vi "ROI Entry Screen_v3.vi"() -> ()   [LabVIEW 2020]
uses:
  Typedefs/Top level VI states.ctl
  ROI Entry screen/Typedefs/ROI move buttons.ctl
  ROI Entry screen/Typedefs/ROI move mode.ctl
  Typedefs/Offsets cluster.ctl
  ROI Entry screen/Typedefs/FGV ROI Time Ops.ctl
  Typedefs/ROI management FG states.ctl
  ROI Entry screen/Typedefs/Redraw ROI.ctl
  ROI Entry screen/Typedefs/ROI Lbox actions.ctl
  ROI Entry screen/SubVIs/Automatic POI detection/Typedefs/Duplicate POI function enum.ctl
  Typedefs/Read Write Enum.ctl
  ROI Entry screen/Typedefs/ROI entry screen ctrl refs cluster.ctl
  Global Variables/General Globals.vi
  User profiles code/Globals/gl_UsrProfiles globals.vi
  ROI Entry screen/Globals/gl_ROI Entry UI globals.vi
  ROI Entry screen/Typedefs/ROI input mode.ctl
panel:
  out "ROI Type":string
  out "Array":bool[](array[boolean])
  in  "Offset ROI":bool
  in  "Arbitrary Plane":bool
  in  "Whole Plane":bool
  in  "Equal Size":bool
  in  "Line Mode":bool
  out "Current ROI Type":string
  out "AOL Z ind. (um)":dbl caption="Motor Z" format="AOL Z   =  %#_g µm"
  in  "Load Reference Image":bool
  out "# POI":i32 format="%.0f ROI"
  in  "Max Z Proj":bool
  out "ROI":T1
  out "Number of lines left":i32 format="%.0f number of lines left"
  in  "Palette Type":T2(ring)
  out "Zplane ind":i32 caption="Z-Plane" format="Z-Plane %.0f"
  in  "Z-Plane Selector":i32(c297)=7
  out "Image Display":T3(plugin-control)
  out "Motor Z ind. (um)":dbl caption="Motor Z" format="Motor Z = %#_g µm"
  out "# of planes":i32 format="# of Planes = %.0f"
  in  "Intensity slider":cluster{i16, i16}(slide)={0, 4095} caption="Intensity" scale=0.0..4095.0
  in  "Channel":enum16{"Green", "Red"}(ring)
  in  "Step size (µm)":u8(slide)=1 min=1 max=100 step=1 scale=1.0..30.0
  in  "ROI offset arrows":T4
  in  "ROI move mode":T5
  in  "Auto Generate":bool
  in  "POI Density":dbl(slide) scale=0.01..1.0
  in  "Tab Control":enum32{"ROI Details", "Folder", "Vaa3D"}(tab)
  in  "Adj. \nMC":bool
  out "Dwell Time (Ind.)":dbl caption="Dwell Time" format="%.2f us"
  out "Laser Power (Ind.)":dbl caption="Laser Power" format="%u %"
  out "Pixel Density (Ind.)":dbl caption="Pixel Density" format="%.2f px/um"
  out "Cycle rate":dbl format="%.2f Hz"
  out "Resolution (Ind.)":dbl caption="Resolution" format="%.2f um/px"
  in  "Laser Power(%)":dbl min=0.0 max=100.0 step=1.0
  in  "Show All":bool
  in  "Delete Lines":bool
  in  "Save ROI File":bool
  in  "ROI LIST":i32[](listbox)
  in  "Rel.  Res.":dbl=1.0 format="%.2g"
  in  "Funct stim.trig.delay (sec)":dbl=0.5 caption="Stimulus trigger delay" min=0.0 max=60.0 step=0.001 format="%#.3fs"
  in  "Enable funct. stimulus":bool caption="Enable stimulus"
  in  "Wavelength (nm)":dbl=920.0 caption="l" min=800.0 max=1080.0 step=1.0 format="%#_g nm"
  in  "Number of Trials":u16=1 caption="Trials" min=1 max=1000 format="%.0f trials"
  in  "Dwell time [us]":dbl=0.1 caption="Scan dwell time\nper pixel (us)" min=0.05 max=20.0 step=0.01 format="%.2f"
  in  "POI dwell time (us)":dbl=4.0 caption="POI dwell time" min=0.05 max=20.0 format="%_3g µs"
  in  "Zoom":dbl=1.0 min=0.001 max=10.0 step=0.1 format="%#.2f x"
  in  "Trial Length (sec)":dbl=1.0 caption="Trial Length" min=0.05 max=60.0 step=1.0 format="%#.3f s"
  in  "Cool-down time (s)":dbl caption="Cool-down time" min=0.0 max=60.0 step=0.05 format="%#.2f s"
  in  "Enable cool-down time":bool caption="Enable stimulus"
  in  "Load ROI File":bool caption="Load\nolder\nPOI"
  in  "Start Plane":i32 caption="From Plane"
  in  "Stop Plane":i32 caption="To Plane"
  in  "Clear All":bool
  in  "Clear Last":bool
  out "Frame Size (Ind.)":dbl caption="Frame Size"
  out "FOV (Ind.)":dbl caption="FOV" format="%d um"
  out "ZPlanes":dbl[][](array[numeric])
  in  "Z-stack folder path":path caption="Experiment folder path"
  in  "spacing_between_points":dbl=10.0 min=0.05 max=100.0 step=1.0 format="%#.3f"
  in  "Call_Vaa3D":bool caption="Load\nolder\nPOI"
  out "Next State":T6=enum."Live Imaging-START"
  in  "Live Imaging":bool
  in  "Acquisition":bool
  in  "Done/Close":bool
  # "ROI Offset"
  # "ROI Removal"
  # "ROI Input"
  # "ROI AutoGen"
  # "Min"
  # "Max"
  # "Plane Filter :"
  # "Original Z Stack Settings"
  # "ROI Input Settings"
  # "Stimulus trigger delay"
  # "Experiment Settings"
  # "Cool-down time"
  # "AOLZ"
  # "Motor Z"
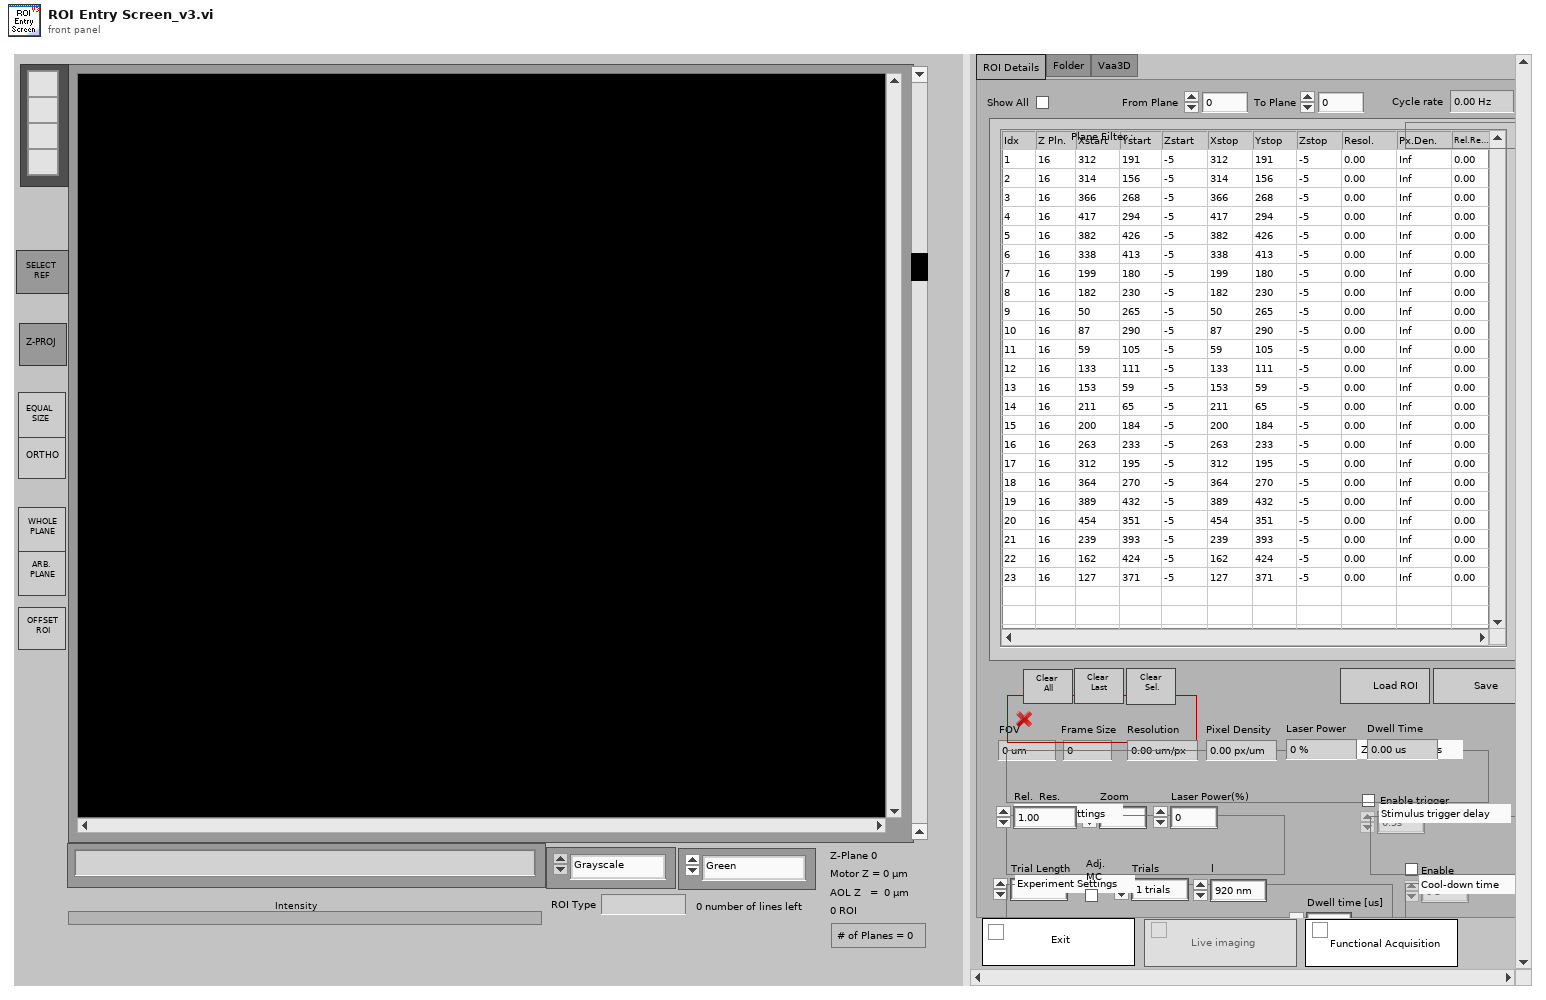
[diagram p1: front panel]
types:
  T1 = cluster{"Global Rectangle":i32[], "Contours":cluster{"Contour Type":u32, "ROI Type":u32, "Points":i32[]}[]}
  T2 = enum16{"Grayscale", "Binary", "Gradient", "Rainbow", "Temperature", "User Defined"}
  T3 = typedef "IMAQ Image.ctl" = refnum<image>
  T4 = typedef "ROI move buttons.ctl" = cluster{"Right":bool, "Left":bool, "Up":bool, "Down":bool, "Up-left":bool, "Up-right":bool, "Down-left":bool, "Down-right":bool}
  T5 = typedef "ROI move mode.ctl" = enum16{"ROI on ALL planes", "ROI on current plane"}
  T6 = typedef "Top level VI states.ctl" = enum16{"None", "Initialise UI", "<STACK PROTOCOL STATES>", "AOL Zstack-START", "AOL Zstack-STOP", "Motor Zstack-START", "Motor Zstack-STOP", "Parameter Sweep-START", "Parameter Sweep-STOP", "<ACQUISITION PROTOCOL STATES> ", "Functional Acquisition-START", "Functional Acquisition-STOP", "Single Plane Acquisition-START", "Single Plane Acquisition-STOP", "Volume Acquisition-START", "Volume Acquisition-STOP", "<LIVE IMAGING PROTOCOL STATES>", "Live Imaging-START", "Live Imaging-STOP", "Live Plane Imaging-START", "Live Plane Imaging-STOP", "Live Volume Imaging-START", "Live Volume Imaging-STOP", "<MOVEMENT CORRECTION PROTOCOL STATES>", "EXIT"}
  T7 = typedef "Offsets cluster.ctl" = cluster{"X offset":i8, "Y offset":i8}
  T8 = cluster{"Load experiment data":refnum<user-event>, "Finish rectangle editing":refnum<user-event>, "Offset all ROI":refnum<user-event>}
  T9 = typedef "ROI info cluster.ctl" = cluster{"Global Rectangle":i32[], "Contours":cluster{"Contour Type":u32, "ROI Type":u32, "Points":i32[]}[]}
  T10 = typedef "FGV ROI Time Ops.ctl" = enum16{"Read", "Write Cycle Time", "Write Cycle Rate"}
  T11 = typedef "Redraw ROI.ctl" = enum16{"Redraw All", "Redraw Deselected", "Draw Last", "Redraw Selected"}
  T12 = typedef "ROI management FG states.ctl" = enum16{"Read", "Write", "Write-from dataset", "Clear Last", "Clear All", "Delete ROI", "Update ROIs time", "Reload last ROI set", "Modify ROI Parameters", "Offset all ROI", "Offset visible ROI", "Modify Dwell Time", "Modify Laser Power"}
  T13 = typedef "ROI Lbox actions.ctl" = enum16{"Idle", "Insert", "Insert_current_plane", "Copy", "Copy_current_plane", "Replicate", "Replicate_current_plane"}
  T14 = typedef "ROI input mode.ctl" = enum16{"Unspecified", "Point-Line-Plane", "Volume"}
  T15 = enum8{"Enabled", "Disabled", "Disabled and Grayed Out"}
  T16 = typedef "Duplicate POI function enum.ctl" = enum16{"Generate", "Adjust number of POI", "Clear register"}
  T17 = typedef "Read Write Enum.ctl" = enum16{"Read", "Write"}
  T18 = typedef "ROI entry screen ctrl refs cluster.ctl" = cluster{"Done button":refnum<vi>, "Imaging button":refnum<vi>, "Acquisition button":refnum<vi>, "Scan dwell time per pixel (us)":refnum<vi>, "# of planes":refnum<vi>, "Zoom Ctrl":refnum<vi>, "Equal size":refnum<vi>, "Channel":refnum<vi>, "Image Display":refnum<vi>, "Z-Plane Selector":refnum<vi>, "Number of lines left":refnum<vi>, "Z-stack folder path":refnum<vi>, "POI Density":refnum<vi>, "Arb Plane Entry":refnum<vi>, "Whole Plane":refnum<vi>, "Line Mode":refnum<vi>, "Clear Last":refnum<vi>, "Clear All":refnum<vi>, "Delete Lines":refnum<vi>, "Trial Length (sec)":refnum<vi>, "Palette Type":refnum<vi>, "Intensity slider":refnum<vi>, "# POI":refnum<vi>, "Max Z Proj":refnum<vi>, "Zplane ind":refnum<vi>, "Wavelength (nm)":refnum<vi>, "Number of Trials":refnum<vi>, "Funct stim.trig.enable":refnum<vi>, "Funct stim.trig.delay (s)":refnum<vi>, "Line Mode":refnum<vi>, "Step size (µm)":refnum<vi>, "ROI move mode":refnum<vi>, "Cool-down time (s)":refnum<vi>, "Enable cool-down time":refnum<vi>, "Motor Z ind. (um)":refnum<vi>, "AOL Z ind. (um)":refnum<vi>, "Load Reference Image":refnum<vi>, "Rel.  Res.":refnum<vi>, "ROI LIST":refnum<vi>, "Show All":refnum<vi>, "ROI Type":refnum<vi>, "Start Plane":refnum<vi>, "Stop Plane":refnum<vi>, "Offset ROI":refnum<vi>, "Tab Control":refnum<vi>, "Laser Power(%)":refnum<vi>, "Cycle rate":refnum<vi>, "FOV (Ind.)":refnum<vi>, "Frame Size (Ind.)":refnum<vi>, "Resolution (Ind.)":refnum<vi>, "Pixel Density (Ind)":refnum<vi>, "Laser Power (Ind.)":refnum<vi>, "Dwell Time (Ind.)":refnum<vi>, "Adj MC":refnum<vi>}
  T19 = typedef "ROI ID Enum.ctl" = enum16{"Point", "MiniScan", "Comp. MiniScan", "Rectangle", "Comp. volume", "Arb. plane point", "None"}
  T20 = typedef "ROI parameters data type.ctl" = cluster{"ROI index":dbl, "ROI ID":dbl, "ROI Time (ns)":dbl, "Pixels in ROI":dbl, "X start":dbl, "Y start":dbl, "Z start":dbl, "X stop":dbl, "Y stop":dbl, "Z stop":dbl, "Angle (deg)":dbl, "Composite ID":dbl, "Number of lines":dbl, "Frame Size":dbl, "Zoom":dbl, "Laser Power (%)":dbl, "ROI group ID":dbl, "Resolution":dbl, "Dwell Time per pixel":dbl, "Pixels per miniscan":dbl, "Original FOV (um)":dbl, "Apparent Frame Size":dbl, "Z Plane Idx":i32[], "Z Plane codes":i32[]}
  T21 = typedef "LVRowAndColumnTypeDef.ctl" = cluster{"Row":i32, "Column":i32}
  T22 = typedef "lveventtype.ctl" = enum32{"Null", "Timeout", "Annotation Menu Selection", "Annotation Menu Selection?", "App Instance Close", "App Instance Close?", "Autoscale Range Change", "Bookmark Info Change", "Cell Edit", "Cell Edit?", "Cursor Grab", "Cursor Grab?", "Cursor Menu Selection", "Cursor Menu Selection?", "Cursor Move", "Cursor Release", "Data Change", "Direction Change", "Display State Change", "Drag Ended", "Drag Enter", "Drag Leave", "Drag Over", "Drag Source Update", "Drag Starting", "Drag Starting?", "Drop", "Exec State Change", "Key Down", "Key Down?", "Key Repeat", "Key Repeat?", "Key Up", "Listbox Double Click", "Menu Activation?", "Menu Selection (App)", "Menu Selection? (App)", "Menu Selection (User)", "Mouse Down", "Mouse Down?", "Mouse Enter", "Mouse Leave", "Mouse Move", "Mouse Up", "Mouse Wheel", "NI Security User Change (App)", "Pane Size", "Panel Close", "Panel Close?", "Panel Resize", "Plot Attribute Change", "Scale Range Change", "Shortcut Menu Activation?", "Shortcut Menu Selection (App)", "Shortcut Menu Selection? (App)", "Shortcut Menu Selection (User)", "Tree Double Click", "Tree Drag", "Tree Drag?", "Tree Drop", "Tree Drop?", "Tree Item Close", "Tree Item Close?", "Tree Item Open", "Tree Item Open?", "User Event", "Value Change"}
  T23 = typedef "ROI Entry screen VI interface 1.ctl" = cluster{"Last Image Display Event info":T24, "ROIs Info []":T25[], "Cancelled":bool, "Done button disabled?":enum8{"Enabled", "Disabled", "Disabled and Grayed Out"}, "Acquisition button disabled?":enum8{"Enabled", "Disabled", "Disabled and Grayed Out"}}
  T24 = typedef "Last Image Display Event info.ctl" = cluster{"Type":i32, "Tool":i32, "Coordinates":i32[], "Other Parameters":sgl[]}
  T25 = typedef "ROI spec.ctl" = cluster{"ROI Enum":T19, "Coordinates":i32[], "Zoom":dbl, "POI Dwell time":dbl, "Rel. Resolution":dbl, "Laser Power":dbl, "Frame Size":dbl, "FOV":dbl, "Z start":dbl, "Z stop":dbl, "Z planeIdx(s)":i32[], "Z planecodes(s)":u8[]}
  T26 = typedef "ROI parameters data type.ctl" = cluster{"ROI index":dbl, "ROI ID":dbl, "ROI Time (ns)":dbl, "Pixels in ROI":dbl, "X start":dbl, "Y start":dbl, "Z start":dbl, "X stop":dbl, "Y stop":dbl, "Z stop":dbl, "Angle (deg)":dbl, "Composite ID":dbl, "Number of lines":dbl, "Frame Size":dbl, "Zoom":dbl, "Laser Power (%)":dbl, "ROI group ID":dbl, "Resolution":dbl, "Dwell Time per pixel":dbl, "Z Plane Idx":i32[], "Z Plane codes":i32[]}
  T27 = typedef "AOL_Globals.ctl" = cluster{"Imaging Protocol":T28, "Number of POI":u16, "Number of Miniscans":u16, "Number of Trials":u16, "Number of Cycles ":u64, "# Averaged Frames":u16, "Laser power (%)":u8, "Pockels (V)":dbl, "Acquisition Length (sec)":dbl, "Fill time (us)":dbl, "POI Dwell time (us)":dbl, "Miniscan Dwell time per pixel (us)":dbl, "PMT 1":dbl, "PMT 2":dbl, "Back Apperture (mA)":dbl, "Frame Size":T29, "Center Frequency":dbl, "Field of View (um)":dbl, "Field of View (norm)":dbl, "DwellTime (us)":dbl, "Ref Dwell Time (us)":dbl, "Wavelength (nm)":dbl, "Zoom":dbl, "AOL Z":dbl, "AOL Mode":T30, "GridXY":dbl, "GridZ":dbl, "TriggerPeriod (sec)":dbl, "Number of Pixels in Miniscan":u16, "Experiment folder path":path, "X centre":dbl, "Y centre":dbl, "Angle (degrees)":dbl, "Angle Xs (degrees)":dbl, "Angle Ys (degrees)":dbl, "Plane Mode":T31, "Threshold":u16[], "Regenerate Chirps":bool, "Rectangle ROI length (pixels)":u16, "Rectangle ROI height (pixels)":u16, "AOD fill":u16, "StartupDelay":i32, "Samples Wait after Trigger":u16, "Slip Cycle":u32, "Add Cycle":bool, "Functional Mode":T32, "Z Start":dbl, "Z Stop":dbl, "# Planes":i32, "Total Pixels":i32, "Variable Miniscan Pixels":u16[], "Use Variable Length":bool, "Use Variable Resolution":bool, "Laser power (%) at Z Start":u8, "Laser power (%) at Z Stop":u8, "Ref Z Step":i8}
  T28 = typedef "Imaging Protocols enum.ctl" = enum16{"AOL Z-Stack", "Motor Z Stack", "Parameter Sweep", "Functional Acquisition", "Single Plane Acquisition", "Volume Acquisition", "Live Imaging", "Live Plane Imaging", "Live Volume Imaging"}
  T29 = typedef "Frame Size.ctl" = u16
  T30 = typedef "AOL modes.ctl" = enum16{"Raster", "Structural", "Pointing", "Mini Scan", "Alignment"}
  T31 = typedef "Plane Mode.ctl" = u16
  T32 = typedef "Functional Mode.ctl" = enum16{"Point", "Line", "Patch", "Plane", "Volume"}
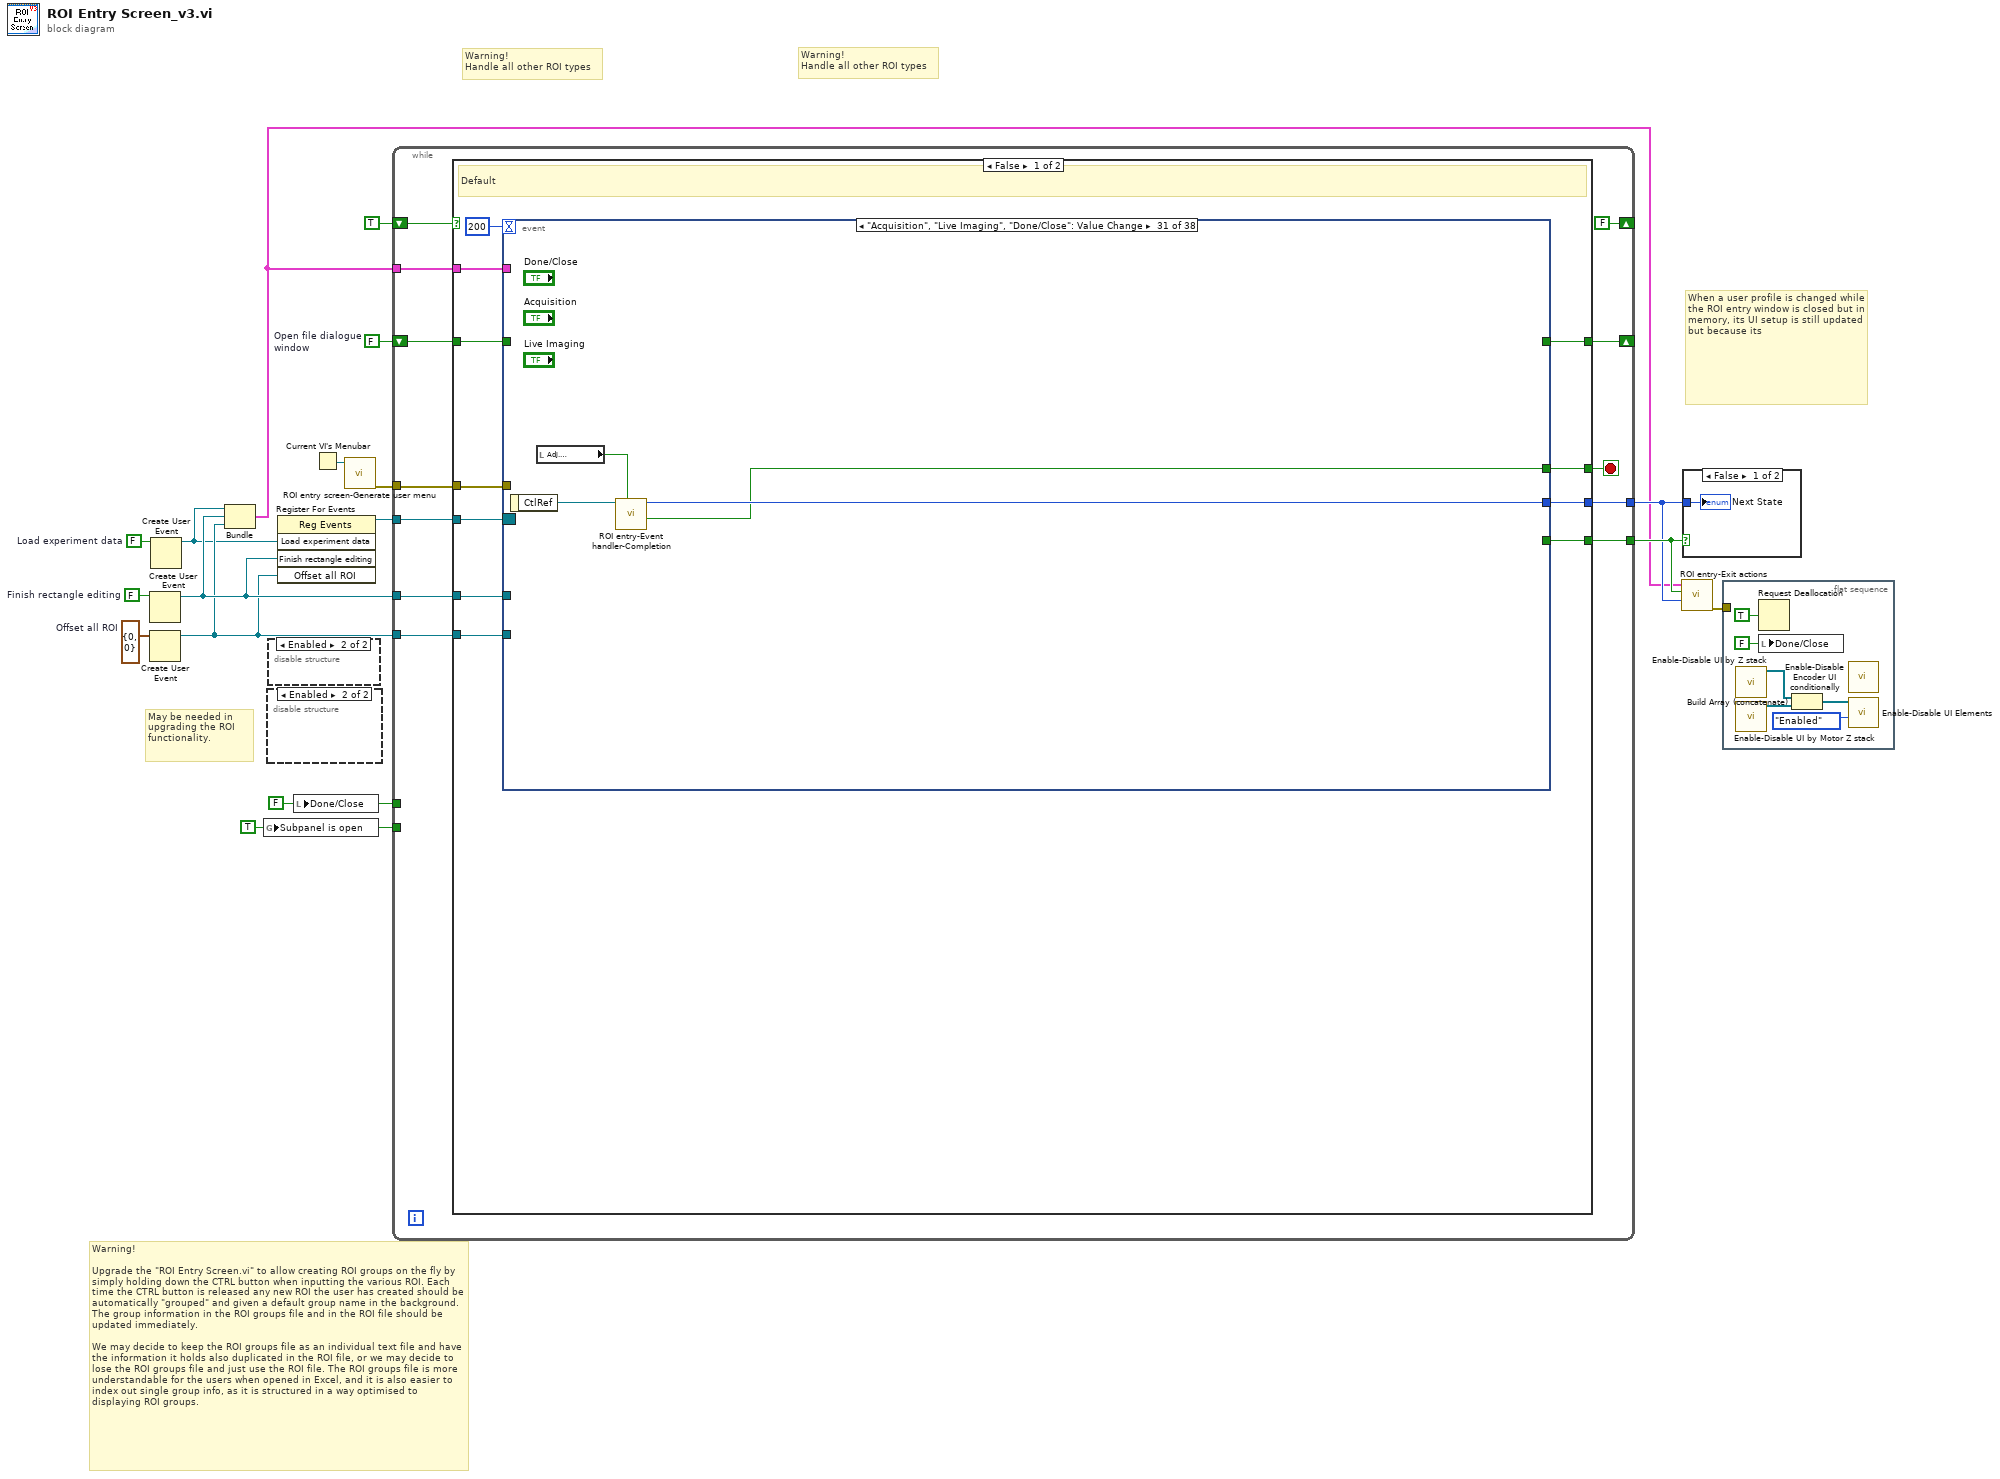
[diagram p0: block diagram]
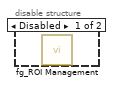
[diagram p2: hidden frame]
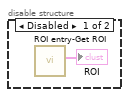
[diagram p3: hidden frame]
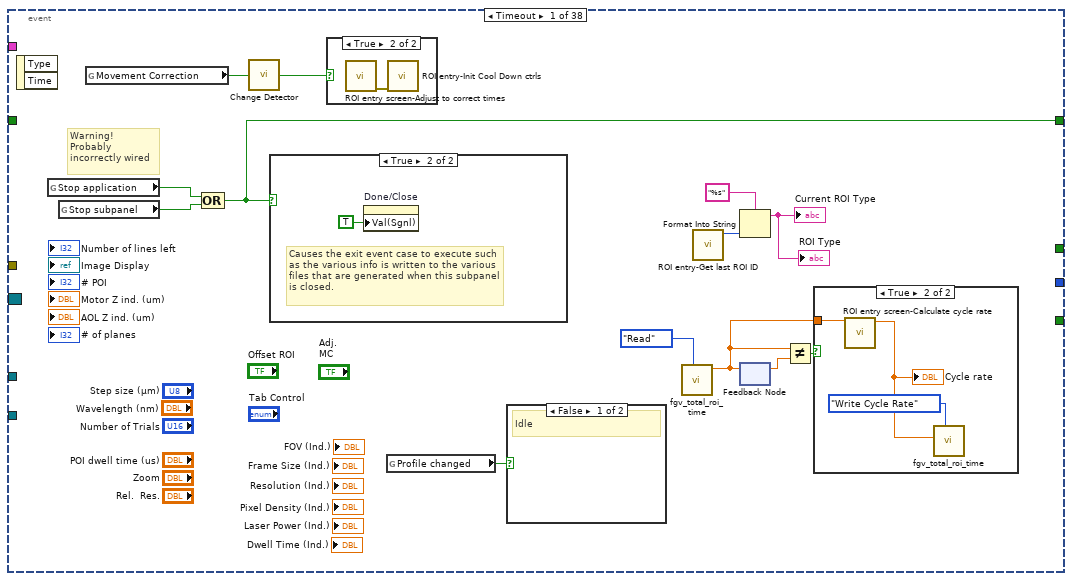
[diagram p5: hidden frame]
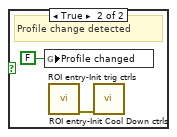
[diagram p7: hidden frame]
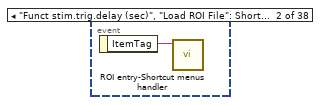
[diagram p10: hidden frame]
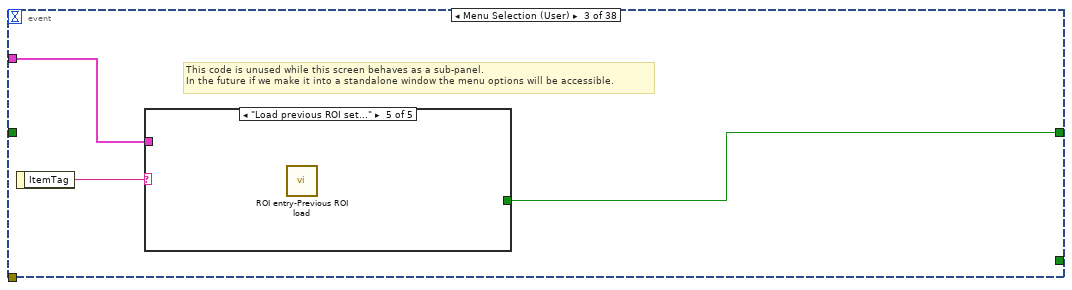
[diagram p11: hidden frame]
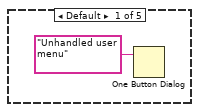
[diagram p12: hidden frame]
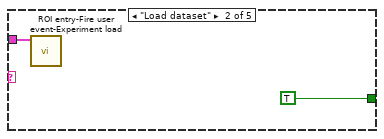
[diagram p13: hidden frame]
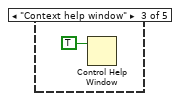
[diagram p14: hidden frame]
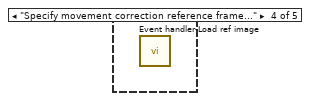
[diagram p15: hidden frame]
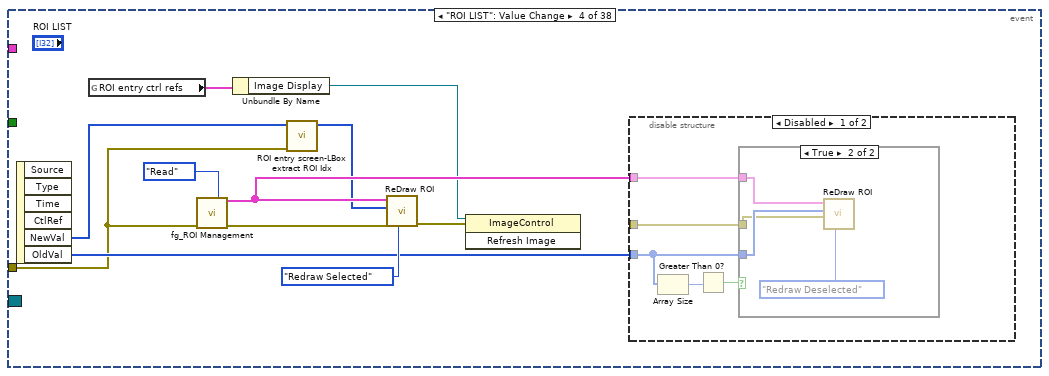
[diagram p16: hidden frame]
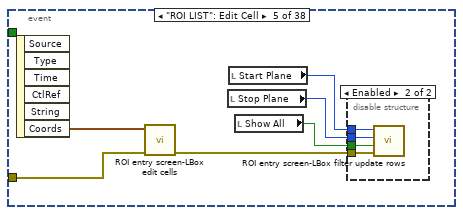
[diagram p19: hidden frame]
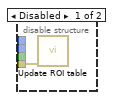
[diagram p20: hidden frame]
diagram:
  w6 = T7 {"X offset"=0, "Y offset"=0}  # Offset all ROI
  w7 = FALSE ("Done/Close")
  w13 = FALSE  # Finish rectangle editing
  w14 = TRUE ("Subpanel is open")
  w15 = FALSE  # Open file dialogue window
  w17 = FALSE  # Load experiment data
  # "When a user profile is changed while the ROI entry window is closed but in memory, its UI setup is still updated but because its"
  # "Warning!\n\nUpgrade the \"ROI Entry Screen.vi\" to allow creating ROI groups on the fly by simply holding down the CTRL button when inputting the various ROI. Each time the CTRL button is released any new ROI the user has created should be automatically \"grouped\" and given a default group name in the background. The group information in the ROI groups file and in the ROI file should be updated immediately.\n\nWe may decide to keep the ROI groups file as an individual text file and have the information it holds also duplicated in the ROI file, or we may decide to lose the ROI groups file and just use the ROI file. The ROI groups file is more understandable for the users when opened in Excel, and it is also easier to index out single group info, as it is structured in a way optimised to displaying ROI groups."
  # "May be needed in upgrading the ROI functionality."
  # "Warning!\nHandle all other ROI types"
  # "Warning!\nHandle all other ROI types"
  n1 = Create User Event(user event datatype=w13) -> (user event=w5:refnum<user-event>)  [unwired: 1 in, 1 out]
  n2 = Create User Event(user event datatype=w6) -> (user event=w4:refnum<user-event>)  [unwired: 1 in, 1 out]
  n3 = Create User Event(user event datatype=w17) -> (user event=w3:refnum<user-event>)  [unwired: 1 in, 1 out]
  n4 = Bundle("Load experiment data"=w3, "Finish rectangle editing"=w5, "Offset all ROI"=w4) -> (w2:T8)  [unwired: 1 in]
  n5 = global write "General Globals.vi" "Subpanel is open"(w14) -> ()
  n6 = disable-structure shown="Enabled" {
    frame Disabled {
      n7 = call "ROI entry-Get ROI.vi"() -> ("ROI info cluster (native format)"=→"ROI":T9)  [unwired: 10 in, 1 out]
    }
    frame Enabled {
    }
  }
  n8 = disable-structure shown="Enabled" {
    frame Disabled {
      n9 = call "fg_ROI Management.vi"() -> ()  [unwired: 6 in, 6 out]
    }
    frame Enabled {
    }
  }
  n10 = register-events(w3, w5, w4) -> (reference out=w16:refnum<event-registration>)  [unwired: 2 in, 1 out]
  n11 = local write "Done/Close"(w7) -> ()
  n12 = Current VI's Menubar() -> (w12:refnum<k9>)
  n13 = call "ROI entry screen-Generate user menu.vi"("Functional Viewer Menu in"=w12) -> ("error out"=w11:errorcluster)  [unwired: 9 in, 1 out]
  n14 = while {
    shift-right: [FALSE] -> _
    shift-left: TRUE -> [w29]
    tunnel: [w27] -> w9
    tunnel: w16 -> [w26]
    tunnel: w2 -> [w25]
    shift-right: [w24] -> _
    shift-left: w15 -> [w23]
    tunnel: w14 -> [_]
    tunnel: w5 -> [w22]
    tunnel: w11 -> [w19]
    tunnel: [w21] -> w10
    tunnel: w7 -> [_]
    tunnel: w4 -> [w20]
    stop <- w30 stop-if-true
    n15 = case shown="False" w29 {
      tunnel: [w40 _] -> w30
      tunnel: [w39 _] -> w27
      tunnel: w26 -> [w38 _]
      tunnel: w25 -> [w37 w312]
      tunnel: [w35 w313] -> w24
      tunnel: w23 -> [w36 _]
      tunnel: w22 -> [w34 _]
      tunnel: [w33 _] -> w21
      tunnel: w20 -> [w32 _]
      tunnel: w19 -> [w31 _]
      frame False {
        # "Default"
        n16 = event shown="[30] \"Acquisition\", \"Live Imaging\", \"Done/Close\": Value Change" {
          selector: w38 -> [_ _ _ _ _ _ _ _ _ _ _ _ _ _ _ _ _ _ _ _ _ _ _ _ _ _ _ _ _ _ _ _ _ _ _ _ _ _]
          dyn-events: _ -> [_ _ _ _ _ _ _ _ _ _ _ _ _ _ _ _ _ _ _ _ _ _ _ _ _ _ _ _ _ _ _ _ _ _ _ _ _ _]
          timeout: 200 -> [_ _ _ _ _ _ _ _ _ _ _ _ _ _ _ _ _ _ _ _ _ _ _ _ _ _ _ _ _ _ _ _ _ _ _ _ _ _]
          tunnel: [_ _ _ _ _ _ _ _ _ _ _ _ _ _ _ _ _ _ _ _ _ _ _ _ _ _ _ _ _ _ w275 _ _ _ _ _ _ w310] -> w40
          tunnel: [_ _ _ _ _ _ _ _ _ _ _ _ _ _ _ _ _ _ _ _ _ _ _ _ _ _ _ _ _ _ w276 _ _ _ _ _ _ _] -> w39
          tunnel: w37 -> [_ _ w64 _ _ _ _ _ _ _ _ _ _ _ _ w197 _ _ _ _ _ _ _ _ _ _ _ _ _ _ _ _ _ _ _ _ _ _]
          tunnel: w36 -> [_ _ _ _ _ _ _ _ _ w157 _ _ _ w188 _ _ _ _ _ _ _ _ _ _ _ _ _ _ _ _ _ _ _ _ _ _ _ _]
          tunnel: [w53 _ w63 _ _ _ _ _ _ _ _ _ _ _ _ _ _ _ _ _ _ _ _ _ _ _ _ _ _ _ _ _ _ _ _ _ _ _] -> w35
          tunnel: w34 -> [_ _ _ _ _ w104 _ _ _ _ _ _ _ _ _ _ _ _ _ _ _ _ _ _ _ _ _ _ _ _ _ _ _ _ _ _ _ _]
          tunnel: [_ _ _ _ _ _ _ _ _ _ _ _ _ _ _ _ _ _ _ _ _ _ _ _ _ _ _ _ _ _ _ _ _ _ _ _ _ w310] -> w33
          tunnel: w32 -> [_ _ _ _ _ _ _ _ _ _ _ w180 _ _ _ _ _ _ _ _ _ _ _ _ _ _ _ _ _ _ _ _ _ _ _ _ _ _]
          tunnel: w31 -> [_ _ _ w72 w94 _ _ _ _ _ _ _ _ _ _ _ _ _ _ _ _ _ _ _ _ w246 _ w269 w270 _ _ _ w289 _ _ _ _ _]
          event Timeout {
            # "Warning!\nProbably\nincorrectly wired"
            n17 = event-data() -> ()  [unwired: 1 in, 2 out]
            n18 = global read "General Globals.vi" "Stop application"() -> (w54:bool)
            n19 = global read "General Globals.vi" "Stop subpanel"() -> (w52:bool)
            n20 = global read "General Globals.vi" "Movement Correction"() -> (w51:bool)
            n21 = Compound Arithmetic op=OR(w54, w52) -> (w53:bool)
            n22 = call <userlib>:"Change Detector.vi"("Value"=w51) -> ("Changed?"=w50:bool)
            n23 = case shown="True" w53 {
              frame False {
              }
              frame True {
                # "Causes the exit event case to execute such as the various info is written to the various files that are generated when this subpanel is closed."
                n24 = property on="Done/Close" class="Bool (strict)"("Val(Sgnl)"=TRUE) -> ()  [unwired: 2 in, 2 out]
              }
            }
            n25 = case shown="True" w50 {
              frame False {
              }
              frame True {
                n26 = call "ROI entry screen-Adjust to correct times.vi"() -> ("error out"=w60:errorcluster)  [unwired: 10 in, 1 out]
                n27 = call "ROI entry-Init Cool Down ctrls.vi"("error in (no error)"=w60) -> ()  [unwired: 10 in, 1 out]
              }
            }
            n28 = global read "gl_UsrProfiles globals.vi" "Profile changed"() -> (w49:bool)
            n29 = case shown="False" w49 {
              frame False {
                # "Idle"
              }
              frame True {
                # "Profile change detected"
                n30 = global write "gl_UsrProfiles globals.vi" "Profile changed"(FALSE ("Profile changed")) -> ()
                n31 = call "ROI entry-Init trig ctrls.vi"() -> ("error out"=w59:errorcluster)  [unwired: 11 in]
                n32 = call "ROI entry-Init Cool Down ctrls.vi"("error in (no error)"=w59) -> ()  [unwired: 10 in, 1 out]
              }
            }
            n33 = call "fgv_total_roi_time.vi"("Op"=FGV_ROI_Time_Ops."Read") -> ("Total cycle time"=w43:dbl)  [unwired: 6 in, 4 out]
            n34 = call "ROI entry-Get last ROI ID.vi"() -> ("ROI ID Enum"=w48:T19)  [unwired: 8 in, 3 out]
            n35 = Format Into String(format string="%s", w48) -> (resulting string=→"Current ROI Type" →"ROI Type":string)  [unwired: 2 in, 1 out]
            n36 = feedback-in #1(w43) -> ()
            n37 = feedback #1() -> (w45:dbl)  [unwired: 1 in]
            n38 = Not Equal?(x=w43, y=w45) -> (x != y?=w44:bool)
            n39 = case shown="True" w44 {
              tunnel: w43 -> [_ w56]
              frame False {
              }
              frame True {
                n40 = call "ROI entry screen-Calculate cycle rate.vi"("Total ROI time"=w56) -> ("Estimated cycle rate"=w57:dbl)  [unwired: 9 in, 1 out]
                "Cycle rate" <- w57
                n41 = call "fgv_total_roi_time.vi"("Op"=FGV_ROI_Time_Ops."Write Cycle Rate", "Cycle Rate"=w57) -> ()  [unwired: 5 in, 5 out]
              }
            }
          }
          event "Funct stim.trig.delay (sec)", "Load ROI File": Shortcut Menu Selection (User) {
            n42 = event-data() -> ("ItemTag"=w62:string)  [unwired: 1 in]
            n43 = call "ROI entry-Shortcut menus handler.vi"("ItemTag"=w62) -> ()  [unwired: 11 in]
          }
          event Menu Selection (User) {
            # "This code is unused while this screen behaves as a sub-panel.\nIn the future if we make it into a standalone window the menu options will be accessible."
            n44 = event-data() -> ("ItemTag"=w65:string)  [unwired: 1 in]
            n45 = case shown="\"Load previous ROI set...\"" w65 {
              tunnel: w64 -> [_ w67 _ _ _]
              tunnel: [_ TRUE _ _ _] -> w63
              frame Default {
                n46 = One Button Dialog(message="Unhandled user menu") -> ()  [unwired: 1 in, 1 out]
              }
              frame "Load dataset" {
                n47 = call "ROI entry-Fire user event-Experiment load.vi"("User Events Cluster"=w67) -> ()  [unwired: 10 in, 1 out]
              }
              frame "Context help window" {
                n48 = Control Help Window(1:TRUE ("Show")) -> ()  [unwired: 1 in]
              }
              frame "Specify movement correction reference frame..." {
                n49 = call "Event handler-Load ref image.vi"() -> ()  [unwired: 10 in, 2 out]
              }
              frame "Load previous ROI set..." {
                n50 = call "ROI entry-Previous ROI load.vi"() -> ()  [unwired: 11 in, 1 out]
              }
            }
          }
          event "ROI LIST": Value Change {
            n51 = event-data() -> ("NewVal"=w70:i32[], "OldVal"=w77:i32[])  [unwired: 1 in, 4 out]
            n52 = global read "gl_ROI Entry UI globals.vi" "ROI entry ctrl refs"() -> (w74:T18)
            n53 = call "fg_ROI Management.vi"("Function"=ROI_management_FG_states."Read", "error in (no error)"=w72) -> ("ROI Setup"=w76:T20[], "error out"=w79:errorcluster)  [unwired: 7 in, 5 out]
            n54 = Unbundle By Name(w74) -> ("Image Display"=w73:refnum<vi>)
            n55 = call "ROI entry screen-LBox extract ROI Idx.vi"("error in (no error)"=w72, "Selected Lines"=w70) -> ("ID"=w71:i32[])  [unwired: 8 in, 1 out]
            n56 = call "ReDraw ROI.vi"("Mode (Redraw All)"=Redraw_ROI."Redraw Selected", "error in"=w79, "Selected/Deselected"=w71, "XYZ Coordinates"=w76) -> ("error out"=w75:errorcluster)  [unwired: 7 in]
            n57 = invoke class="ImageControl" method="Refresh Image"(reference=w73, error in=w75) -> ()  [unwired: 1 in, 3 out]
            n58 = disable-structure shown="Disabled" {
              disable-tunnel: w77 -> [w85 _]
              disable-tunnel: _ -> [w82 _]
              disable-tunnel: w76 -> [w81 _]
              frame Disabled {
                n59 = Array Size(array=w85) -> (size(s)=w84:i32)
                n60 = Greater Than 0?(x=w84) -> (x > 0?=w83:bool)
                n61 = case shown="True" w83 {
                  tunnel: w85 -> [_ w89]
                  tunnel: w82 -> [_ w88]
                  tunnel: w81 -> [_ w87]
                  frame False {
                  }
                  frame True {
                    n62 = call "ReDraw ROI.vi"("Mode (Redraw All)"=Redraw_ROI."Redraw Deselected", "error in"=w88, "Selected/Deselected"=w89, "XYZ Coordinates"=w87) -> ()  [unwired: 7 in, 1 out]
                  }
                }
              }
              frame Enabled {
              }
            }
          }
          event "ROI LIST": Edit Cell {
            n63 = event-data() -> ("Coords"=w95:T21)  [unwired: 1 in, 5 out]
            n64 = call "ROI entry screen-LBox edit cells.vi"("error in (no error)"=w94, "Selected Cell"=w95) -> ("error out"=w90:errorcluster)  [unwired: 9 in]
            n65 = local read "Stop Plane"() -> (w92:i32)
            n66 = local read "Start Plane"() -> (w93:i32)
            n67 = local read "Show All"() -> (w91:bool)
            n68 = disable-structure shown="Enabled" {
              disable-tunnel: w90 -> [w96 w100]
              disable-tunnel: w93 -> [_ w99]
              disable-tunnel: w92 -> [_ w98]
              disable-tunnel: w91 -> [_ w97]
              frame Disabled {
                n69 = call "Update ROI table.vi"("error in (no error)"=w96) -> ()  [unwired: 10 in, 1 out]
              }
              frame Enabled {
                n70 = call "ROI entry screen-LBox filter update rows.vi"("error in (no error)"=w100, "Show All"=w97, "Stop Plane"=w98, "Start Plane"=w99) -> ()  [unwired: 6 in, 2 out]
              }
            }
          }
          event Key Down; Key Up {
            n71 = event-data() -> ("ScanCode"=w103:i16, "Type"=w102:T22)  [unwired: 1 in]
            n72 = case shown="\"Key Down\"" w102 {
              tunnel: w104 -> [_ w109]
              tunnel: w103 -> [w105 w108]
              tunnel: [w105 i16 -1 ("ScanCode")] -> w101
              frame "Key Down" {
              }
              frame "Key Up", Default {
                n73 = global read "gl_ROI Entry UI globals.vi" "Rectangle being edited"() -> (w107:bool)
                n74 = case shown="True" w107 {
                  tunnel: w108 -> [_ w112]
                  tunnel: w109 -> [_ w111]
                  frame False {
                  }
                  frame True {
                    w113 = i16 30  # 30 is the "A" key
                    # "Rectangle being edited"
                    n75 = Equal?(x=w112, y=w113) -> (x = y?=w110:bool)
                    n76 = case shown="True" w110 {
                      tunnel: w111 -> [_ w115]
                      frame False {
                      }
                      frame True {
                        # "The \"A\" key has just been released"
                        n77 = Generate User Event(user event=w115, event data cluster=FALSE ("event data")) -> ()  [unwired: 2 in, 2 out]
                      }
                    }
                  }
                }
              }
            }
            n78 = global write "gl_ROI Entry UI globals.vi" "Pressed key ScanCode"(w101) -> ()
          }
          event "Image Display": Mouse Up; User Event {
            # "Adjusts the Experiment Time and Cool-down time value to the theoretical calculated values which result from the fact that the acquisition time is always an integer multiple of the cycle time."
            n79 = event-data() -> ("Type"=w123:u32)  [unwired: 1 in]
            n80 = call "ROI entry-User ROI event-Analyse.vi"("Event Type"=w123) -> ("error out"=w121:errorcluster, "output cluster"=w122:T23)  [unwired: 9 in]
            n81 = call "ROI entry-User ROI event-Apply new ROI.vi"("error in (no error)"=w121, "Input cluster"=w122) -> ("error IO"=w120:errorcluster)  [unwired: 9 in]
            n82 = call "ROI entry screen-Adjust to correct times.vi"("error in (no error)"=w120) -> ("error out"=w116:errorcluster)  [unwired: 9 in, 1 out]
            n83 = local read "Stop Plane"() -> (w118:i32)
            n84 = local read "Start Plane"() -> (w119:i32)
            n85 = local read "Show All"() -> (w117:bool)
            n86 = disable-structure shown="Enabled" {
              disable-tunnel: w116 -> [w124 w128]
              disable-tunnel: w119 -> [_ w127]
              disable-tunnel: w118 -> [_ w126]
              disable-tunnel: w117 -> [_ w125]
              frame Disabled {
                n87 = call "Update ROI table.vi"("error in (no error)"=w124) -> ()  [unwired: 10 in, 1 out]
              }
              frame Enabled {
                n88 = call "ROI entry screen-LBox filter update rows.vi"("error in (no error)"=w128, "Show All"=w125, "Stop Plane"=w126, "Start Plane"=w127) -> ()  [unwired: 6 in, 2 out]
              }
            }
          }
          event "ROI LIST": Shortcut Menu Selection (User) {
            n89 = event-data() -> ("ItemTag"=w134:string)  [unwired: 1 in, 7 out]
            n90 = To Lower Case(string=w134) -> (all lower case string=w133:string)
            n91 = To Lower Case(string=string[] ["Insert ", "Insert_current_plane", "Copy", "Copy_current_plane", "Replicate", "Replicate_current_plane"]) -> (all lower case string=w140:string[])
            n92 = Search 1D Array(1D array=w140, element=w133) -> (index of element=w139:i32)  [unwired: 1 in]
            n93 = case shown="0..5" w139 {
              selector: w139 -> [_ w151]
              tunnel: [ROI_Lbox_actions."Idle" ("ROI LBox Actions") w150] -> w135
              frame -1, Default {
              }
              frame 0..5 {
                # "Insert"
                n94 = Increment(x=w151) -> (x+1=w149:i32)
                n95 = To Word Integer(number=w149) -> (16bit integer=w148:i16)
                n96 = Type Cast(type=ROI_Lbox_actions."Replicate_current_plane" ("ROI LBox Actions"), x=w148) -> (*(type *) &x=w150:T13)
              }
            }
            n97 = call "ROI entry screen-LBox shortcut actions.vi"("ROI LBox Actions"=w135) -> ("error out"=w131:errorcluster, "ROI Info"=w130:T23)  [unwired: 9 in]
            n98 = call "ROI entry-User ROI event-Apply new ROI.vi"("error in (no error)"=w131, "Input cluster"=w130) -> ("error IO"=w132:errorcluster)  [unwired: 9 in]
            n99 = call "ROI entry screen-Adjust to correct times.vi"("error in (no error)"=w132) -> ("error out"=w129:errorcluster)  [unwired: 9 in, 1 out]
            n100 = local read "Stop Plane"() -> (w137:i32)
            n101 = local read "Start Plane"() -> (w138:i32)
            n102 = local read "Show All"() -> (w136:bool)
            n103 = disable-structure shown="Enabled" {
              disable-tunnel: w129 -> [w142 w143]
              disable-tunnel: w138 -> [_ w146]
              disable-tunnel: w137 -> [_ w145]
              disable-tunnel: w136 -> [_ w144]
              frame Disabled {
                n104 = call "Update ROI table.vi"("error in (no error)"=w142) -> ()  [unwired: 10 in, 1 out]
              }
              frame Enabled {
                n105 = call "ROI entry screen-LBox filter update rows.vi"("error in (no error)"=w143, "Show All"=w144, "Stop Plane"=w145, "Start Plane"=w146) -> ()  [unwired: 6 in, 2 out]
              }
            }
          }
          event Value Change {
            n106 = event-data() -> ()  [unwired: 1 in, 1 out]
            n107 = call "ROI entry-Offset mode colour.vi"() -> ()  [unwired: 11 in, 1 out]
          }
          event User Event {
            n108 = event-data() -> ()  [unwired: 1 in, 1 out]
            n109 = case shown="True" w157 {
              tunnel: [w161 w176] -> w158
              tunnel: [w159 w175] -> w156
              tunnel: [w160 w174] -> w155
              frame False {
                # "Do not open file dialogue window"
                n110 = local read "Z-stack folder path"() -> (w162:path)
                n111 = Empty String/Path?(string/path=w162) -> (empty?=w166:bool)
                n112 = call <vilib>:"Check if File or Folder Exists.vi"("path"=w162) -> ("file or folder exists?"=w164:bool)  [unwired: 8 in, 2 out]
                n113 = Not(x=w164) -> (.not. x?=w165:bool)
                n114 = Or(x=w166, y=w165) -> (x .or. y?=w163:bool)
                n115 = case shown="True" w163 {
                  tunnel: w162 -> [w167 _]
                  tunnel: [w167 w171] -> w161
                  tunnel: [_ w170] -> w160
                  tunnel: [_ w169] -> w159
                  frame False {
                  }
                  frame True {
                    n116 = call "File Dialog3"("prompt"="Please specify a valid experiment folder", "button label"="Load") -> ("selected path"=w171:path, "cancelled"=w169:bool, "error out"=w170:errorcluster)  [unwired: 10 in, 1 out]
                  }
                }
              }
              frame True {
                # "Open file dialogue window"
                n117 = call "File Dialog2"("prompt"="Please specify a valid experiment folder", "button label"="Load") -> ("selected path"=w176:path, "cancelled"=w175:bool, "error out"=w174:errorcluster)  [unwired: 10 in, 1 out]
              }
            }
            n118 = Empty String/Path?(string/path=w158) -> (empty?=w154:bool)
            n119 = Compound Arithmetic op=OR(w154, w156, w155) -> (w153:bool)
            n120 = case shown="False" w153 {
              tunnel: w158 -> [w178 _]
              frame False {
                # "File path is valid"
                n121 = local write "Z-stack folder path"(w178) -> ()
                n122 = call "ROI entry-Load dataset.vi"("Experiment folder path OR Z-stack folder path"=w178) -> ()  [unwired: 10 in, 1 out]
              }
              frame True {
                # "Empty file path / Not a path / User cancelled / Error"
              }
            }
          }
          event User Event {
            # "Functionality temporarily disabled"
            n123 = event-data() -> ()  [unwired: 1 in, 2 out]
          }
          event Value Change {
            n124 = event-data() -> ("NewVal"=w179:T4)  [unwired: 1 in]
            n125 = call "ROI entry-Event handler-ROI offset.vi"("Offset all ROI-User Event in"=w180, "ROI offset arrows: NewVal"=w179) -> ()  [unwired: 9 in, 1 out]
          }
          event "Call_Vaa3D": Value Change {
            n126 = event-data() -> ()  [unwired: 1 in, 6 out]
            n127 = local read "Z-stack folder path"() -> (w181:path)
            n128 = call "Call Vaa3D.vi"("spacing_between_points"="spacing_between_points", "Call_Vaa3D"="Call_Vaa3D", "Z-stack folder path"=w181) -> ()  [unwired: 8 in, 1 out]
          }
          event "Load ROI File": Value Change {
            # "Adjusts the Experiment Time and Cool-down time value to the theoretical calculated values which result from the fact that the acquisition time is always an integer multiple of the cycle time."
            n129 = event-data() -> ()  [unwired: 1 in, 1 out]
            n130 = flat-sequence {
              tunnel: [w190] -> w189
              tunnel: w188 -> [_]
              tunnel: w189 -> [_]
              tunnel: [w191] -> w184
              tunnel: w187 -> [w195]
              tunnel: w186 -> [w193]
              tunnel: w185 -> [w192]
              tunnel: w184 -> [w194]
              frame #0 {
                n131 = call "ROI entry-Previous ROI load.vi"() -> ("Proceed"=w190:bool)  [unwired: 11 in]
              }
              frame #1 {
                n132 = call "ROI entry screen-Adjust to correct times.vi"() -> ("error out"=w191:errorcluster)  [unwired: 10 in, 1 out]
              }
              frame #2 {
                n133 = call "ROI entry screen-LBox filter update rows.vi"("error in (no error)"=w194, "Show All"=w192, "Stop Plane"=w193, "Start Plane"=w195) -> ()  [unwired: 6 in, 2 out]
              }
            }
            n134 = local read "Start Plane"() -> (w187:i32)
            n135 = local read "Stop Plane"() -> (w186:i32)
            n136 = local read "Show All"() -> (w185:bool)
          }
          event "Line Mode": Value Change {
            n137 = event-data() -> ()  [unwired: 1 in, 5 out]
            n138 = call "fgv_ROI equal size line coords.vi"("Function"=enum16{"Intialize", "Write", "Read", "Clear"}."Clear") -> ()  [unwired: 9 in, 2 out]
          }
          event "Z-stack folder path": Value Change {
            n139 = event-data() -> ()  [unwired: 1 in, 1 out]
            n140 = call "ROI entry-Fire user event-Experiment load.vi"("User Events Cluster"=w197) -> ()  [unwired: 10 in, 1 out]
          }
          event "Z-Plane Selector": Value Change {
            w200 = FALSE ("Max Z Proj")
            # "Max Z-projection button automatically released when the scrollbar is moved."
            # "Compensates for Labview bug."
            n141 = event-data() -> ()  [unwired: 1 in, 1 out]
            n142 = property on="Z-Plane Selector" class="Scroll (strict)"() -> ("DocMax"=w206:dbl, "DocMin"=w205:dbl)  [unwired: 2 in, 2 out]
            n143 = feedback-in #2("Z-Plane Selector") -> ()
            n144 = feedback #2() -> (w207:i32)  [unwired: 1 in]
            n145 = Decrement(x=w206) -> (x-1=w201:dbl)
            n146 = property on="Z-Plane Selector" class="Scroll (strict)"() -> ("PageSize"=w199:dbl)  [unwired: 2 in, 2 out]
            n147 = local write "Max Z Proj"(w200) -> ()
            n148 = Less?(x="Z-Plane Selector", y=w205) -> (x < y?=w204:bool)
            n149 = Greater?(x="Z-Plane Selector", y=w201) -> (0:w203:bool)
            n150 = feedback #3() -> (w198:dbl)  [unwired: 1 in]
            n151 = feedback-in #3(w199) -> ()
            n152 = Or(x=w203, y=w204) -> (x .or. y?=w202:bool)
            n153 = case shown="False" w202 {
              tunnel: w207 -> [_ w214]
              tunnel: "Z-Plane Selector" -> [w209 _]
              tunnel: w200 -> [_ _]
              tunnel: w198 -> [_ w215]
              frame False {
                # "Input value is in range"
                n154 = flat-sequence {
                  tunnel: w209 -> [w210]
                  frame #0 {
                    "Zplane ind" <- w210
                  }
                  frame #1 {
                    n155 = local read "ROI LIST"() -> (w211:i32[])
                    n156 = call "ROI entry-Handle ROI change.vi"("Selected ROI"=w211, "ROI management"=ROI_management_FG_states."Read") -> ("error out"=w212:errorcluster)  [unwired: 7 in, 2 out]
                    n157 = call "ROI entry-Index Zplane position.vi"("error in (no error)"=w212) -> ()  [unwired: 9 in, 2 out]
                  }
                }
              }
              frame True {
                # "Prevents out of range inputs"
                n158 = property on="Z-Plane Selector" class="Scroll (strict)"("PageSize"=w215) -> ()  [unwired: 2 in, 2 out]
                n159 = call "ROI entry-Set Z-plane selector.vi"("Z-plane selector value"=w214) -> ()  [unwired: 10 in, 1 out]
              }
            }
          }
          event "Channel", "Max Z Proj": Value Change {
            n160 = event-data() -> ()  [unwired: 1 in, 1 out]
            n161 = call "ROI entry-Event handler-Max projection.vi"() -> ()  [unwired: 11 in, 1 out]
          }
          event "Intensity slider": Value Change {
            n162 = event-data() -> ()  [unwired: 1 in, 1 out]
            n163 = call "ROI entry-Set display mapping.vi"() -> ()  [unwired: 11 in, 1 out]
          }
          event "Palette Type": Value Change {
            n164 = event-data() -> ("NewVal"=w216:T2)  [unwired: 1 in]
            n165 = call "ROI entry-Set palette type.vi"("Palette:Palette Type"=w216) -> ()  [unwired: 10 in, 1 out]
          }
          event "Arbitrary Plane": Value Change {
            n166 = event-data() -> ()  [unwired: 1 in, 6 out]
            n167 = call "ROI entry-Event handler-Arb entry.vi"() -> ()  [unwired: 11 in, 1 out]
          }
          event "Whole Plane": Value Change {
            n168 = event-data() -> ()  [unwired: 1 in, 6 out]
            n169 = call "ROI entry-Event handler-Whole plane.vi"() -> ()  [unwired: 12 in]
          }
          event "Equal Size": Value Change {
            n170 = event-data() -> ()  [unwired: 1 in, 6 out]
            n171 = call "ROI entry-Event handler-Equal Size.vi"() -> ()  [unwired: 12 in]
          }
          event "Auto Generate": Value Change {
            n172 = event-data() -> ()  [unwired: 1 in, 1 out]
            n173 = disable-structure shown="Disabled" {
              frame Disabled {
                n174 = call "fg_ROI Management.vi"("Function"=ROI_management_FG_states."Read") -> ("ROI Setup"=w220:T26[])  [unwired: 5 in, 5 out]
                n175 = Empty Array?(array=w220) -> (empty?=w219:bool)
                n176 = case shown="False" w219 {
                  tunnel: [w239 w242] -> w218
                  frame False {
                    # "User-specified ROIs exist"
                    n177 = Two Button Dialog(message="WARNING\n\nThe Auto-generate function will overwrite existing ROIs.\n", 2:"Proceed..." ("T button name (\"OK\")")) -> (T button?=w239:bool)  [unwired: 1 in]
                  }
                  frame True {
                    w242 = TRUE  # Proceed
                    # "No user-specified ROIs"
                  }
                }
                n178 = case shown="True" w218 {
                  frame False {
                  }
                  frame True {
                    n179 = call "POI Autogen number entry window.vi"() -> ("Cancelled"=w221:bool, "Number of POI"=w222:i32)  [unwired: 10 in]
                    n180 = case shown="False" w221 {
                      tunnel: w222 -> [w234 _]
                      frame False {
                        w232 = TRUE
                        w237 = T15."Enabled" ("Disabled")
                        # "Not cancelled. Auto-generate POIs."
                        n181 = global read "gl_ROI Entry UI globals.vi" "ROI entry ctrl refs"() -> (w228:T18)
                        n182 = call "fg_ROI Management.vi"("Function"=ROI_management_FG_states."Clear All") -> ("error out"=w227:errorcluster)  [unwired: 5 in, 5 out]
                        n183 = call "ROI entry-Clear ROI overlay.vi"("error in (no error)"=w227) -> ("Image Out"=w226:T3)  [unwired: 9 in, 1 out]
                        n184 = Unbundle By Name(w228) -> ("Image Display"=w229:refnum<vi>)
                        n185 = call "Auto generate POIs.vi"("Number of POI to generate"=w234, "Image refnum in"=w226) -> ("POI Array"=w235:T25[], "Number of POI generated"=w236:i32)  [unwired: 8 in]
                        n186 = call "ROI entry-Get selected Z-plane index.vi"() -> ("Z-plane selector (index)"=w225:i32)  [unwired: 10 in, 1 out]
                        n187 = global write "gl_ROI Entry UI globals.vi" "Input Mode"(ROI_input_mode."Point-Line-Plane" ("t")) -> ()
                        n188 = Initialize Array(w225, w236) -> (w224:i32[])
                        n189 = property class="ImageControl"(reference=w229, "Line Tool Button Visible"=w232, "Point Tool Button Visible"=w232) -> ()  [unwired: 1 in, 2 out]
                        n190 = call "ROI entry screen-main buttons management.vi"("Acquisition button boolean text"="Functional Acquisition" ("Boolean Text.Text"), "Imaging button disabled?"=T15."Disabled and Grayed Out" ("Disabled"), "Acquisition button disabled?"=w237, "Done button disabled?"=w237) -> ()  [unwired: 8 in]
                        n191 = call "Apply ROIs.vi"("Mode (Redraw All)"=enum16{"Redraw All", "Draw Last"}."Redraw All", "ROIs Info []"=w235, 11:w224) -> ()  [unwired: 6 in, 3 out]
                      }
                      frame True {
                        # "Cancelled"
                      }
                    }
                  }
                }
              }
              frame Enabled {
                n192 = call "POI Gen Engine.vi"("Function"=Duplicate_POI_function_enum."Generate") -> ()  [unwired: 10 in, 1 out]
              }
            }
          }
          event "POI Density": Value Change {
            n193 = event-data() -> ()  [unwired: 1 in, 1 out]
            n194 = global read "General Globals.vi" "First autogen"() -> (w244:bool)
            n195 = case shown="False" w244 {
              frame False {
                n196 = call "POI Gen Engine.vi"("Function"=Duplicate_POI_function_enum."Adjust number of POI") -> ()  [unwired: 10 in, 1 out]
              }
              frame True {
              }
            }
          }
          event "Clear All": Value Change {
            n197 = event-data() -> ()  [unwired: 1 in, 6 out]
            n198 = flat-sequence {
              tunnel: w246 -> [w247]
              tunnel: [w247] -> _
              frame #0 {
                n199 = call "ROI entry-Event handler-Clear All ROI.vi"() -> ()  [unwired: 12 in]
              }
            }
          }
          event "Clear Last": Value Change {
            # "WARNING!\nMore work may be needed"
            n200 = event-data() -> ()  [unwired: 1 in, 6 out]
            n201 = call "ROI entry-Get last ROI ID.vi"() -> ("error out"=w252:errorcluster, "NO ROI"=w251:bool, "ROI ID Enum"=w250:T19)  [unwired: 8 in, 1 out]
            n202 = call "ROI entry-Handle ROI change.vi"("error in (no error)"=w252, "ROI management"=ROI_management_FG_states."Clear Last" ("Function")) -> ("error out"=w249:errorcluster, "No ROI"=w254:bool, "Number of ROI"=w253:i32)  [unwired: 7 in]
            n203 = case shown="False" w254 {
              tunnel: w253 -> [w257 _]
              tunnel: w251 -> [_ w262]
              tunnel: w250 -> [_ w261]
              tunnel: w249 -> [w256 w260]
              tunnel: [w256 w260] -> w248
              frame False {
                # "Some ROI exist"
                n204 = local read "Arbitrary Plane"() -> (w258:bool)
                n205 = case shown="True" w258 {
                  tunnel: w257 -> [w259 _]
                  frame True {
                    # "Arb. Plane Entry mode is active"
                    n206 = call "ROI entry screen-Arb plane UI setup.vi"("Number of ROI"=w259) -> ()  [unwired: 11 in]
                  }
                  frame False {
                    # "Arb. Plane Entry mode is not active"
                  }
                }
              }
              frame True {
                # "No ROIs specified"
                n207 = case shown="False" w262 {
                  tunnel: w261 -> [w264 _]
                  frame False {
                    n208 = call "ROI entry-Set ROI tool on Clear All.vi"("Last ROI ID Enum"=w264) -> ()  [unwired: 10 in, 1 out]
                  }
                  frame True {
                  }
                }
                n209 = call "ROI entry-Actions on all ROI cleared.vi"("No ROIs (T)"=TRUE ("empty?")) -> ()  [unwired: 11 in]
              }
            }
            n210 = call "ROI entry screen-Adjust to correct times.vi"("error in (no error)"=w248) -> ()  [unwired: 9 in, 2 out]
          }
          event "Show All", "Start Plane", "Stop Plane": Value Change {
            n211 = event-data() -> ()  [unwired: 1 in, 6 out]
            n212 = call "ROI entry screen-LBox filter update rows.vi"("error in (no error)"=w269, "Show All"="Show All", "Stop Plane"="Stop Plane", "Start Plane"="Start Plane") -> ("Array"=→"Array":bool[])  [unwired: 6 in, 1 out]
          }
          event "Delete Lines": Value Change {
            n213 = event-data() -> ()  [unwired: 1 in, 6 out]
            n214 = flat-sequence {
              tunnel: w270 -> [w271]
              frame #0 {
                n215 = call "ROI entry screen-LBox delete rows.vi"("error in (no error)"=w271) -> ()  [unwired: 10 in, 1 out]
              }
            }
          }
          event "Save ROI File": Value Change {
            n216 = event-data() -> ()  [unwired: 1 in, 6 out]
            n217 = call "fgv_AOL_Globals Read.vi"() -> ("AOL_Globals"=w273:T27)  [unwired: 9 in, 2 out]
            n218 = Unbundle By Name(w273) -> ("Experiment folder path"=w272:path)
            n219 = call "ROI entry screen-Update ROI and save to ROI file.vi"("Experiment folder path"=w272) -> ()  [unwired: 9 in, 2 out]
          }
          event "Acquisition", "Live Imaging", "Done/Close": Value Change {
            n220 = event-data() -> ("CtlRef"=w277:refnum<vi>)  [unwired: 1 in]
            n221 = local read "Adj. \nMC"() -> (w274:bool)
            n222 = call "ROI entry-Event handler-Completion.vi"("Adj Timing for MC"=w274, "Ctrl ref of the control that caused the user event"=w277) -> ("Exit"=w275:bool, "Imaging Mode"=w276:T6)  [unwired: 8 in]
          }
          event "Dwell time [us]", "Trial Length (sec)": Value Change {
            # "Adjusts the Experiment Time and Cool-down time value to the theoretical calculated values which result from the fact that the acquisition time is always an integer multiple of the cycle time."
            n223 = event-data() -> ()  [unwired: 1 in, 1 out]
            n224 = call "Limit entered trial length.vi"() -> ("error out"=w288:errorcluster)  [unwired: 11 in]
            n225 = call "fg_ROI Management.vi"("Dwell Time [us]"="Dwell time [us]", "Function"=ROI_management_FG_states."Modify Dwell Time", "error in (no error)"=w288) -> ("Total ROI time"=w285:dbl, "error out"=w286:errorcluster)  [unwired: 6 in, 5 out]
            n226 = call "fgv_total_roi_time.vi"("Op"=FGV_ROI_Time_Ops."Write Cycle Time", "error in (no error)"=w286, "Total cycle time"=w285) -> ("error out"=w283:errorcluster)  [unwired: 4 in, 4 out]
            n227 = call "fgv_AOL_Globals Read.vi"("error in (no error)"=w283) -> ("error out"=w282:errorcluster, "AOL_Globals"=w281:T27)  [unwired: 8 in, 1 out]
            n228 = Bundle By Name(cluster=w281, "POI Dwell time (us)"="Dwell time [us]", "Miniscan Dwell time per pixel (us)"="Dwell time [us]") -> (w279:T27)
            n229 = call "fgv_AOL_Globals Write.vi"("error in (no error)"=w282, "AOL_Globals"=w279) -> ("error out"=w280:errorcluster)  [unwired: 9 in]
            n230 = call "ROI entry screen-Adjust to correct times.vi"("error in (no error)"=w280) -> ()  [unwired: 9 in, 2 out]
          }
          event "Laser Power(%)": Value Change {
            n231 = event-data() -> ()  [unwired: 1 in, 6 out]
            n232 = call "ROI entry screen-LBox update laser power.vi"("error in (no error)"=w289, "Laser Power %"="Laser Power(%)") -> ()  [unwired: 9 in, 1 out]
          }
          event "Load Reference Image": Value Change {
            # "This button is needed in the ROI entry screen because the equivalent button in the main software panel is disabled while the ROI screen is open (to prevent certain errors which could otherwise occur due to unhandled combinations of UI interaction)."
            n233 = event-data() -> ()  [unwired: 1 in, 1 out]
            n234 = flat-sequence {
              tunnel: [w292] -> w291
              tunnel: w291 -> [w293]
              frame #0 {
                n235 = global read "General Globals.vi" "Movement Correction"() -> (w292:bool)
              }
              frame #1 {
                n236 = call "Event handler-Load ref image.vi"() -> ("error out"=w296:errorcluster, "Error or cancelled"=w295:bool)  [unwired: 10 in]
                n237 = Compound Arithmetic op=OR(w295, w296) -> (w294:bool)
                n238 = case shown="False" w294 {
                  tunnel: w293 -> [w297 _]
                  frame False {
                    # "Ref selected"
                    n239 = case shown="False" w297 {
                      frame False {
                        # "MC was OFF"
                        n240 = global read "gl_ROI Entry UI globals.vi" "ROI entry ctrl refs"() -> (w301:T18)
                        n241 = Unbundle By Name(w301) -> ("Acquisition button"=w302:refnum<vi>)
                        n242 = property on="Property Node" class="Bool"(reference=w302, "DisabledEnum"=2) -> (error out=w298:errorcluster)  [unwired: 1 in, 1 out]
                        n243 = call "fgv_Enforce AOL Z repeat.vi"("Function"=Read_Write_Enum."Write", "Enforce AOL Z repeat"=TRUE) -> ()  [unwired: 8 in, 2 out]
                        n244 = flat-sequence {
                          tunnel: w298 -> [_]
                          frame #0 {
                            n245 = call "Message Window.vi"("Message string"="NOTE\nMovement correction has been automatically enabled.\n\nRepeat the AOL Z-stack with movement correction before you can proceed to functional acquisition.\n") -> ()  [unwired: 10 in, 1 out]
                          }
                        }
                      }
                      frame True {
                      }
                    }
                  }
                  frame True {
                    # "Cancelled or error"
                  }
                }
              }
            }
          }
          event "Enable funct. stimulus", "Funct stim.trig.delay (sec)": Value Change {
            n246 = event-data() -> ()  [unwired: 1 in, 1 out]
            n247 = flat-sequence {
              frame #0 {
                # "Prevents entering trigger delays <1ms"
                n248 = Greater Or Equal?(x="Funct stim.trig.delay (sec)", y=0.001) -> (x >= y?=w307:bool)
                n249 = Select(t="Funct stim.trig.delay (sec)", s=w307, f=0.0) -> (s? t:f=w306:dbl)
                n250 = local write "Funct stim.trig.delay (sec)"(w306) -> ()
              }
              frame #1 {
                n251 = call "Stimulus trigger delay event handler.vi"() -> ()  [unwired: 12 in]
              }
            }
          }
          event "Cool-down time (s)", "Enable cool-down time": Value Change {
            # "Adjusts the Experiment Time and Cool-down time value to the theoretical calculated values which result from the fact that the acquisition time is always an integer multiple of the cycle time."
            n252 = event-data() -> ()  [unwired: 1 in, 1 out]
            n253 = call "ROI entry screen-Adjust to correct times.vi"() -> ()  [unwired: 10 in, 2 out]
          }
          event "Funct stim.trig.delay (sec)", "Enable funct. stimulus": Mouse Enter {
            # "Stops the \"Stimulus trigger delay\" control blinking if blinking was triggered."
            n254 = event-data() -> ()  [unwired: 1 in, 1 out]
            n255 = call "ROI entry-Stop trig delay blinking.vi"() -> ()  [unwired: 12 in]
          }
          event Panel Close {
            w310 = TRUE ("Stop loop")
            n256 = event-data() -> ()  [unwired: 1 in, 1 out]
          }
        }
      }
      frame True {
        # "Initialisation"
        n257 = flat-sequence {
          tunnel: w312 -> [w370]
          tunnel: [w370] -> w311
          tunnel: w311 -> [w381]
          tunnel: [w382] -> w313
          frame #0 {
            n258 = control-ref of="ROI LIST"() -> (w338:refnum<vi>)
            n259 = control-ref of="Image Display"() -> (w358:refnum<vi>)
            n260 = control-ref of="Tab Control"() -> (w325:refnum<vi>)
            n261 = control-ref of="Z-Plane Selector"() -> (w355:refnum<vi>)
            n262 = control-ref of="Delete Lines"() -> (w316:refnum<vi>)
            n263 = control-ref of="Adj. MC"() -> (w314:refnum<vi>)
            n264 = control-ref of="Arbitrary Plane"() -> (w335:refnum<vi>)
            n265 = control-ref of="Line Mode"() -> (w333:refnum<vi>)
            n266 = control-ref of="Clear Last"() -> (w337:refnum<vi>)
            n267 = control-ref of="Clear All"() -> (w336:refnum<vi>)
            n268 = control-ref of="Offset ROI"() -> (w328:refnum<vi>)
            n269 = control-ref of="Done/Close"() -> (w348:refnum<vi>)
            n270 = control-ref of="Live Imaging"() -> (w349:refnum<vi>)
            n271 = control-ref of="Acquisition"() -> (w350:refnum<vi>)
            n272 = control-ref of="Equal Size"() -> (w332:refnum<vi>)
            n273 = control-ref of="Max Z Proj"() -> (w365:refnum<vi>)
            n274 = control-ref of="Line Mode"() -> (w331:refnum<vi>)
            n275 = control-ref of="Enable funct. stimulus"() -> (w345:refnum<vi>)
            n276 = control-ref of="Enable cool-down time"() -> (w343:refnum<vi>)
            n277 = control-ref of="Load Reference Image"() -> (w339:refnum<vi>)
            n278 = control-ref of="Show All"() -> (w330:refnum<vi>)
            n279 = control-ref of="Whole Plane"() -> (w334:refnum<vi>)
            n280 = control-ref of="# of planes"() -> (w352:refnum<vi>)
            n281 = control-ref of="FOV (Ind.)"() -> (w322:refnum<vi>)
            n282 = control-ref of="Frame Size (Ind.)"() -> (w321:refnum<vi>)
            n283 = control-ref of="Resolution (Ind.)"() -> (w320:refnum<vi>)
            n284 = control-ref of="Dwell Time (Ind.)"() -> (w317:refnum<vi>)
            n285 = control-ref of="Start Plane"() -> (w327:refnum<vi>)
            n286 = control-ref of="Stop Plane"() -> (w326:refnum<vi>)
            n287 = control-ref of="Laser Power(%)"() -> (w324:refnum<vi>)
            n288 = control-ref of="Cycle rate"() -> (w323:refnum<vi>)
            n289 = control-ref of="Pixel Density (Ind.)"() -> (w319:refnum<vi>)
            n290 = control-ref of="Laser Power (Ind.)"() -> (w318:refnum<vi>)
            n291 = control-ref of="Dwell time [us]"() -> (w351:refnum<vi>)
            n292 = control-ref of="Number of lines left"() -> (w356:refnum<vi>)
            n293 = control-ref of="Trial Length (sec)"() -> (w360:refnum<vi>)
            n294 = control-ref of="# POI"() -> (w363:refnum<vi>)
            n295 = control-ref of="Zplane ind"() -> (w366:refnum<vi>)
            n296 = control-ref of="Wavelength (nm)"() -> (w367:refnum<vi>)
            n297 = control-ref of="Number of Trials"() -> (w368:refnum<vi>)
            n298 = control-ref of="Funct stim.trig.delay (sec)"() -> (w369:refnum<vi>)
            n299 = control-ref of="Cool-down time (s)"() -> (w344:refnum<vi>)
            n300 = control-ref of="Motor Z ind. (um)"() -> (w342:refnum<vi>)
            n301 = control-ref of="AOL Z ind. (um)"() -> (w341:refnum<vi>)
            n302 = control-ref of="Rel.  Res."() -> (w315:refnum<vi>)
            n303 = control-ref of="Zoom"() -> (w353:refnum<vi>)
            n304 = control-ref of="Channel"() -> (w354:refnum<vi>)
            n305 = control-ref of="Palette Type"() -> (w361:refnum<vi>)
            n306 = control-ref of="ROI move mode"() -> (w346:refnum<vi>)
            n307 = control-ref of="ROI Type"() -> (w329:refnum<vi>)
            n308 = control-ref of="Z-stack folder path"() -> (w357:refnum<vi>)
            n309 = control-ref of="POI Density"() -> (w359:refnum<vi>)
            n310 = control-ref of="Intensity slider"() -> (w362:refnum<vi>)
            n311 = control-ref of="Step size (µm)"() -> (w347:refnum<vi>)
            n312 = Bundle By Name(cluster=T18 {"Done button"=refnum, "Imaging button"=refnum, "Acquisition button"=refnum, "Scan dwell time per pixel (us)"=refnum, "# of planes"=refnum, "Zoom Ctrl"=refnum, "Equal size"=refnum, "Channel"=refnum, "Image Display"=refnum, "Z-Plane Selector"=refnum, "Number of lines left"=refnum, "Z-stack folder path"=refnum, "POI Density"=refnum, "Arb Plane Entry"=refnum, "Whole Plane"=refnum, "Line Mode"=refnum, "Clear Last"=refnum, "Clear All"=refnum, "Delete Lines"=refnum, "Trial Length (sec)"=refnum, "Palette Type"=refnum, "Intensity slider"=refnum, "# POI"=refnum, "Max Z Proj"=refnum, "Zplane ind"=refnum, "Wavelength (nm)"=refnum, "Number of Trials"=refnum, "Funct stim.trig.enable"=refnum, "Funct stim.trig.delay (s)"=refnum, "Line Mode"=refnum, "Step size (µm)"=refnum, "ROI move mode"=refnum, "Cool-down time (s)"=refnum, "Enable cool-down time"=refnum, "Motor Z ind. (um)"=refnum, "AOL Z ind. (um)"=refnum, "Load Reference Image"=refnum, "Rel.  Res."=refnum, "ROI LIST"=refnum, "Show All"=refnum, "ROI Type"=refnum, "Start Plane"=refnum, "Stop Plane"=refnum, "Offset ROI"=refnum, "Tab Control"=refnum, "Laser Power(%)"=refnum, "Cycle rate"=refnum, "FOV (Ind.)"=refnum, "Frame Size (Ind.)"=refnum, "Resolution (Ind.)"=refnum, "Pixel Density (Ind)"=refnum, "Laser Power (Ind.)"=refnum, "Dwell Time (Ind.)"=refnum, "Adj MC"=refnum} ("Ctrl refs cluster"), "Done button"=w348, "Imaging button"=w349, "Acquisition button"=w350, "Scan dwell time per pixel (us)"=w351, "# of planes"=w352, "Zoom Ctrl"=w353, "Equal size"=w332, "Channel"=w354, "Image Display"=w358, "Z-Plane Selector"=w355, "Number of lines left"=w356, "Z-stack folder path"=w357, "POI Density"=w359, "Arb Plane Entry"=w335, "Line Mode"=w333, "Clear Last"=w337, "Clear All"=w336, "Delete Lines"=w316, "Trial Length (sec)"=w360, "Palette Type"=w361, "Intensity slider"=w362, "# POI"=w363, "Max Z Proj"=w365, "Zplane ind"=w366, "Line Mode"=w331, "Whole Plane"=w334, "Wavelength (nm)"=w367, "Number of Trials"=w368, "Funct stim.trig.enable"=w345, "Funct stim.trig.delay (s)"=w369, "Step size (µm)"=w347, "ROI move mode"=w346, "Cool-down time (s)"=w344, "Enable cool-down time"=w343, "Motor Z ind. (um)"=w342, "AOL Z ind. (um)"=w341, "Load Reference Image"=w339, "Rel.  Res."=w315, "ROI LIST"=w338, "Show All"=w330, "ROI Type"=w329, "Start Plane"=w327, "Stop Plane"=w326, "Offset ROI"=w328, "Tab Control"=w325, "Laser Power(%)"=w324, "Cycle rate"=w323, "FOV (Ind.)"=w322, "Frame Size (Ind.)"=w321, "Resolution (Ind.)"=w320, "Pixel Density (Ind)"=w319, "Laser Power (Ind.)"=w318, "Dwell Time (Ind.)"=w317, "Adj MC"=w314) -> (w364:T18)
            n313 = global write "gl_ROI Entry UI globals.vi" "ROI entry ctrl refs"(w364) -> ()
          }
          frame #1 {
            n314 = control-ref of="Pane"() -> (w380:refnum<vi>)
            n315 = control-ref of="Pane 2"() -> (w379:refnum<vi>)
            n316 = call "ZSliceCompute.vi"("Function"=Read_Write_Enum."Read") -> ("AOL Z Planes(um)"=w373:dbl[], "Motor Z Planes(um)"=w374:dbl[])  [unwired: 7 in, 2 out]
            n317 = Build Array(w380, w379) -> (w378:refnum<vi>[])
            n318 = Build Array(w374, w373) -> (w372:dbl[][])
            n319 = call "ROI entry-Initialisation.vi"("Pane refs array"=w378, "User Events Cluster"=w381) -> ("Open file dialogue window"=w382:bool)  [unwired: 9 in]
            n320 = call "fgv_Enforce AOL Z repeat.vi"("Function"=Read_Write_Enum."Write", "Enforce AOL Z repeat"=FALSE) -> ()  [unwired: 8 in, 2 out]
            n321 = Transpose 2D Array(2D array=w372) -> (transposed array=→"ZPlanes":dbl[][])
          }
        }
      }
    }
  }
  n322 = call "ROI entry-Exit actions.vi"("Imaging Mode"=w9, "Stop loop"=w10, "User Events cluster"=w2) -> ("error out"=w8:errorcluster)  [unwired: 8 in]
  n323 = case shown="False" w10 {
    tunnel: w9 -> [w383 _]
    frame False {
      "Next State" <- w383
    }
    frame True {
    }
  }
  n324 = flat-sequence {
    tunnel: w8 -> [_]
    frame #0 {
      n325 = call "Enable-Disable UI by Z stack.vi"() -> ("Controls refs to enable/disable"=w386:refnum<vi>[])  [unwired: 11 in]
      n326 = call "Enable-Disable UI by Motor Z stack.vi"() -> ("Controls to disable"=w384:refnum<vi>[])  [unwired: 11 in]
      n327 = Request Deallocation(TRUE ("flag")) -> ()
      n328 = local write "Done/Close"(FALSE ("Done/Close")) -> ()
      n329 = Build Array (concatenate)(w386, w384) -> (w385:refnum<vi>[])
      n330 = call "Enable-Disable Encoder UI conditionally.vi"() -> ()  [unwired: 11 in, 1 out]
      n331 = call "Enable-Disable UI Elements.vi"("Enable/Disable"=T15."Enabled", "Ctrl ref's"=w385) -> ()  [unwired: 9 in, 1 out]
    }
  }
